vi "Change Alias.vi"() -> ()   [LabVIEW 2019]
uses:
  <vilib>/httpClient/POSTBuffer.vi
  <vilib>/httpClient/LabVIEWHTTPClient.lvlib
panel:
  out "error out":errorcluster
  in  "Minion ID":string="cRIO-9068--SN-1856EBC--MAC-00-80-2F-14-B6-CD"
  in  "Server":string="http://localhost"
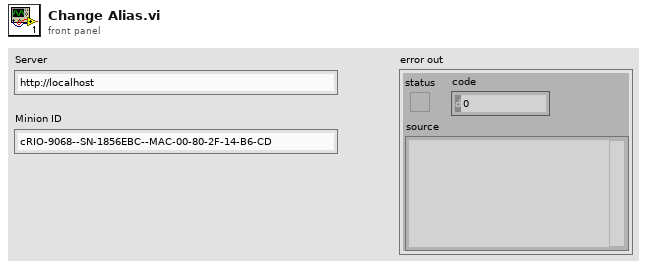
[diagram p1: front panel]
types:
  T1 = typedef "LabVIEWHTTPClient.lvlib/ClientHandle.ctl" = refnum<k1>
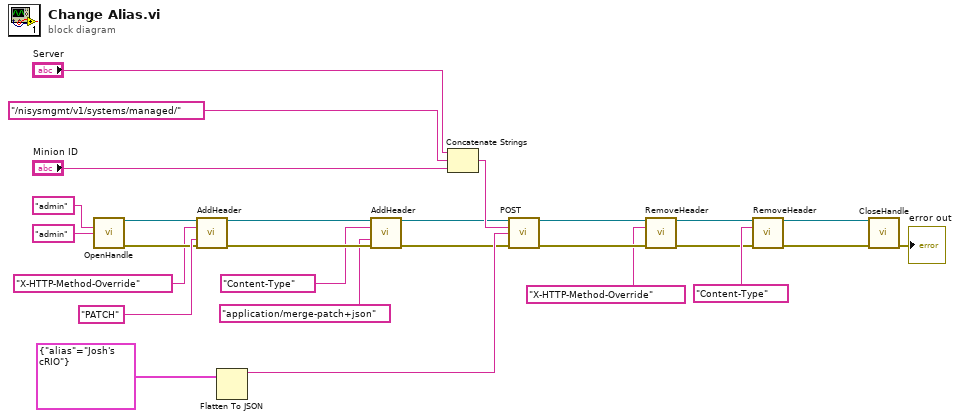
[diagram p0: block diagram]
diagram:
  n1 = call <vilib>:"OpenHandle.vi"("username"="admin", "password"="admin") -> ("client handle out"=w26:T1, "error out"=w25:errorcluster)  [unwired: 12 in]
  n2 = call <vilib>:"AddHeader.vi"("client handle"=w26, "header"="X-HTTP-Method-Override", "value"="PATCH", "error in (no error)"=w25) -> ("client handle out"=w11:T1, "error out"=w12:errorcluster)  [unwired: 10 in]
  n3 = Flatten To JSON(anything=cluster{"alias":string} {"alias"="Josh's cRIO"}) -> (JSON string=w14:string)  [unwired: 2 in, 1 out]
  n4 = call <vilib>:"AddHeader.vi"("client handle"=w11, "header"="Content-Type", "value"="application/merge-patch+json", "error in (no error)"=w12) -> ("client handle out"=w10:T1, "error out"=w9:errorcluster)  [unwired: 10 in]
  n5 = Concatenate Strings("Server", "/nisysmgmt/v1/systems/managed/" ("url"), "Minion ID") -> (w16:string)
  n6 = call-poly <vilib>:"POST.vi"("client handle"=w10, "url"=w16, "buffer"=w14, "error in (no error)"=w9) -> ("client handle out"=w24:T1, "error out"=w23:errorcluster)  [unwired: 8 in, 2 out]
  n7 = call <vilib>:"RemoveHeader.vi"("client handle"=w24, "header"="X-HTTP-Method-Override", "error in (no error)"=w23) -> ("client handle out"=w5:T1, "error out"=w3:errorcluster)  [unwired: 11 in]
  n8 = call <vilib>:"RemoveHeader.vi"("client handle"=w5, "header"="Content-Type", "error in (no error)"=w3) -> ("client handle out"=w1:T1, "error out"=w2:errorcluster)  [unwired: 11 in]
  n9 = call <vilib>:"CloseHandle.vi"("client handle"=w1, "error in (no error)"=w2) -> ("error out"=→"error out":errorcluster)  [unwired: 13 in]
